vi "Grabber Position to Angles.vi"(8 "Backarm Length":dbl, 9 "Forearm Length":dbl, 10 "Y Initial":dbl, 11 "X Initial":dbl) -> (0 "Forearm Angle\nDegrees 2":dbl format="%.2f", 1 "Backarm Angle\nDegrees 2":dbl format="%.2f", 2 "Forearm Angle\nDegrees 1":dbl format="%.2f", 3 "Backarm Angle\nDegrees 1":dbl format="%.2f")   [LabVIEW 2017]
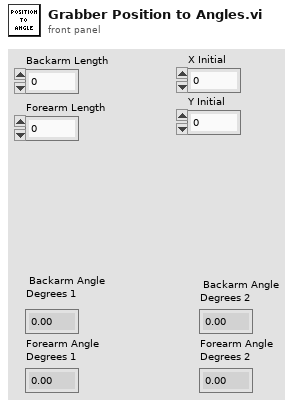
[diagram p1: front panel]
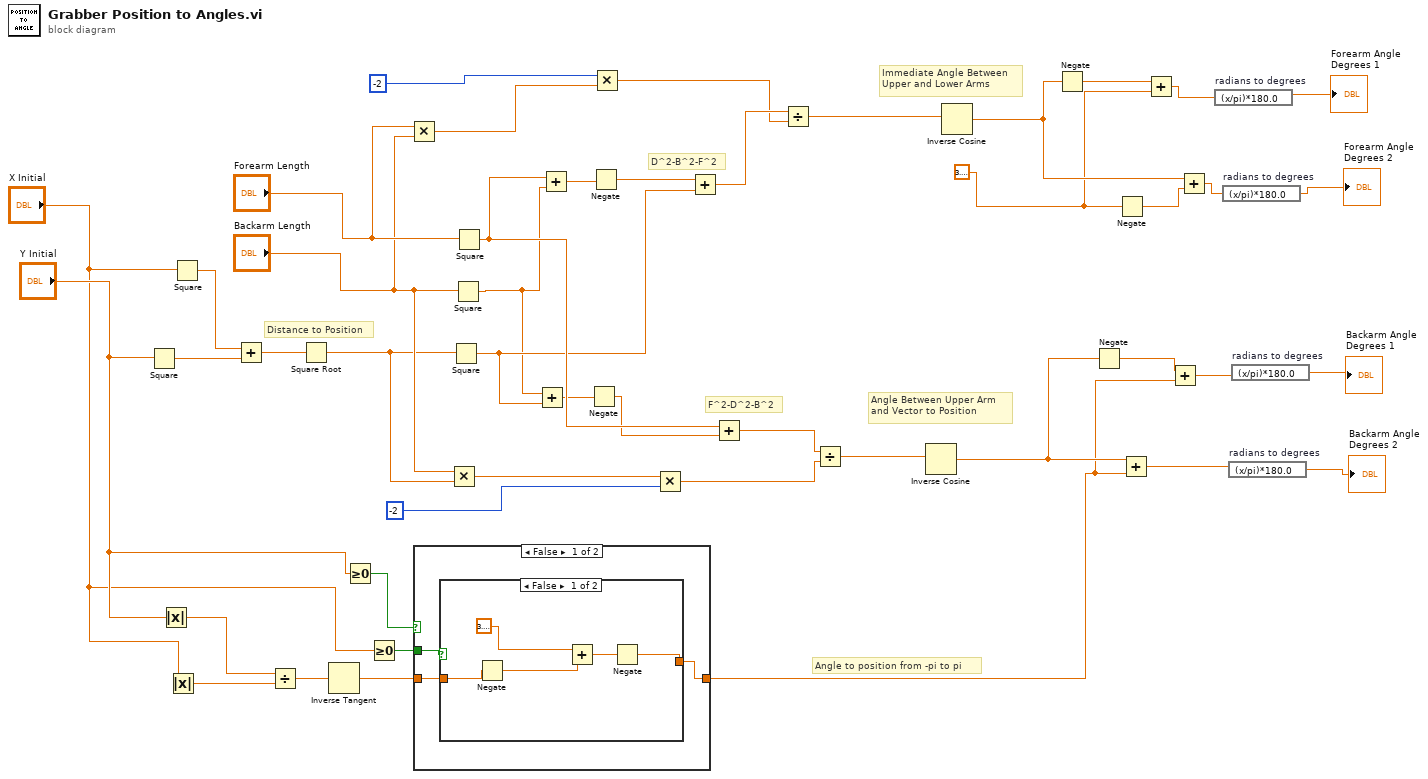
[diagram p0: block diagram]
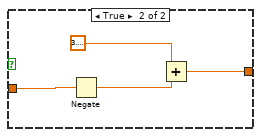
[diagram p2: hidden frame]
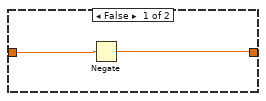
[diagram p4: hidden frame]
diagram:
  w21 = 3.141592653589793
  # "Angle Between Upper Arm\nand Vector to Position"
  # "Immediate Angle Between\nUpper and Lower Arms"
  # "F^2-D^2-B^2"
  # "D^2-B^2-F^2"
  # "Distance to Position"
  # "Angle to position from -pi to pi"
  n1 = Square(x="Y Initial") -> (x^2=w45:dbl)
  n2 = Absolute Value(x="Y Initial") -> (abs(x)=w11:dbl)
  n3 = Absolute Value(x="X Initial") -> (abs(x)=w10:dbl)
  n4 = Square(x="X Initial") -> (x^2=w46:dbl)
  n5 = Add(x=w46, y=w45) -> (x+y=w44:dbl)
  n6 = Divide(x=w11, y=w10) -> (x/y=w9:dbl)
  n7 = Square Root(x=w44) -> (sqrt(x)=w41:dbl)
  n8 = Inverse Tangent(1:w9) -> (0:w2:dbl)
  n9 = Greater Or Equal To 0?(x="Y Initial") -> (x >= 0?=w7:bool)
  n10 = Greater Or Equal To 0?(x="X Initial") -> (x >= 0?=w5:bool)
  n11 = Multiply(x="Forearm Length", y="Backarm Length") -> (x*y=w40:dbl)
  n12 = case shown="False" w7 {
    tunnel: w5 -> [w49 w61]
    tunnel: w2 -> [w48 w60]
    tunnel: [w47 w59] -> w1
    frame False {
      n13 = case shown="False" w49 {
        tunnel: w48 -> [w52 w58]
        tunnel: [w50 w55] -> w47
        frame False {
          n14 = Negate(x=w52) -> (-x=w54:dbl)
          n15 = Add(x=3.141592653589793, y=w54) -> (x+y=w51:dbl)
          n16 = Negate(x=w51) -> (-x=w50:dbl)
        }
        frame True {
          n17 = Negate(x=w58) -> (-x=w56:dbl)
          n18 = Add(x=3.141592653589793, y=w56) -> (x+y=w55:dbl)
        }
      }
    }
    frame True {
      n19 = case shown="True" w61 {
        tunnel: w60 -> [w63 w64]
        tunnel: [w62 w64] -> w59
        frame False {
          n20 = Negate(x=w63) -> (-x=w62:dbl)
        }
        frame True {
        }
      }
    }
  }
  n21 = Multiply(x="Backarm Length", y=w41) -> (x*y=w37:dbl)
  n22 = Square(x=w41) -> (x^2=w33:dbl)
  n23 = Square(x="Backarm Length") -> (x^2=w32:dbl)
  n24 = Square(x="Forearm Length") -> (x^2=w34:dbl)
  n25 = Add(x=w32, y=w33) -> (x+y=w30:dbl)
  n26 = Add(x=w34, y=w32) -> (x+y=w36:dbl)
  n27 = Negate(x=w30) -> (-x=w31:dbl)
  n28 = Negate(x=w36) -> (-x=w35:dbl)
  n29 = Multiply(x=-2, y=w40) -> (x*y=w28:dbl)
  n30 = Multiply(x=w37, y=-2) -> (x*y=w26:dbl)
  n31 = Add(x=w35, y=w33) -> (x+y=w29:dbl)
  n32 = Add(x=w34, y=w31) -> (x+y=w27:dbl)
  n33 = Divide(x=w29, y=w28) -> (x/y=w25:dbl)
  n34 = Divide(x=w27, y=w26) -> (x/y=w24:dbl)
  n35 = Inverse Cosine(1:w24) -> (0:w4:dbl)
  n36 = Inverse Cosine(1:w25) -> (0:w23:dbl)
  n37 = Negate(x=w23) -> (-x=w22:dbl)
  n38 = Negate(x=w4) -> (-x=w3:dbl)
  n39 = Negate(x=w21) -> (-x=w20:dbl)
  n40 = Add(x=w4, y=w1) -> (x+y=w12:dbl)
  n41 = Add(x=w22, y=w21) -> (x+y=w19:dbl)
  n42 = Add(x=w3, y=w1) -> (x+y=w15:dbl)
  n43 = Add(x=w23, y=w20) -> (x+y=w17:dbl)
  n44 = expression code="(x/pi)*180.0" "radians to degrees"(w19) -> (→"Forearm Angle\nDegrees 1":dbl)
  n45 = expression code="(x/pi)*180.0" "radians to degrees"(w17) -> (→"Forearm Angle\nDegrees 2":dbl)
  n46 = expression code="(x/pi)*180.0" "radians to degrees"(w12) -> (→"Backarm Angle\nDegrees 2":dbl)
  n47 = expression code="(x/pi)*180.0" "radians to degrees"(w15) -> (→"Backarm Angle\nDegrees 1":dbl)
